vi "Check If Line Exists.vi"(8 "error in":errorcluster, 10 "Name to Locate":string, 11 "SQLite configuration in":refnum<class "SQLite configuration.lvclass">) -> (0 "error out":errorcluster, 1 "Index":i32, 2 "Line out":T1, 3 "SQLite configuration out":refnum<class "SQLite configuration.lvclass">, 5 "Found?":bool)   [LabVIEW 2014, in "SQLite configuration.lvclass"]
doc: "Checks if a line already exists within a configuration."
uses:
  SQLite configuration.lvclass
  Line.ctl
  <vilib>/NI/Tag Bus Module Framework/channel/TBM channel.lvclass
  SQLite configuration.lvclass/SQLite configuration.ctl
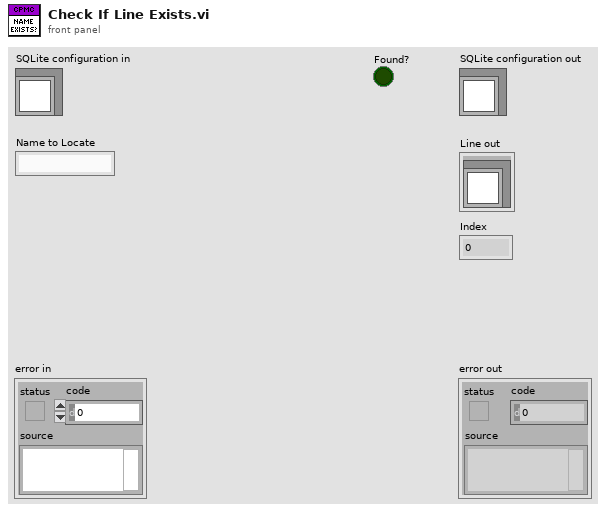
[diagram p1: front panel]
types:
  T1 = typedef "SQLite configuration.lvclass/Line.ctl" = cluster{"channel":refnum<class "TBM channel.lvclass">}
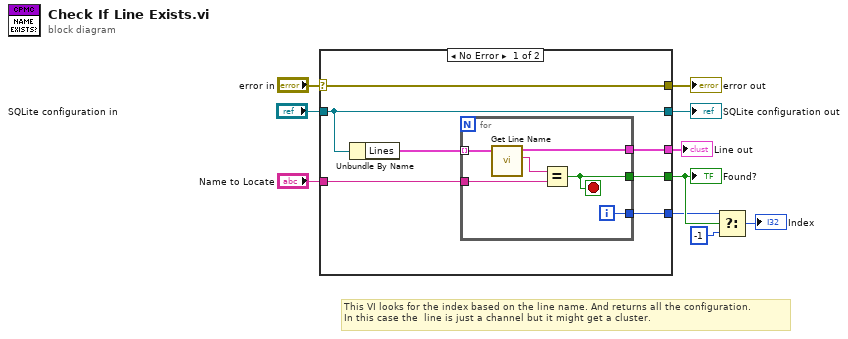
[diagram p0: block diagram]
diagram:
  # "This VI looks for the index based on the line name. And returns all the configuration. \nIn this case the  line is just a channel but it might get a cluster."
  n1 = case shown="No Error" "error in" {
    selector: "error in" -> [w17 w25]
    tunnel: [w17 w25] -> w9
    tunnel: [w16 w24] -> w7
    tunnel: "SQLite configuration in" -> [w16 w24]
    tunnel: "Name to Locate" -> [w14 _]
    tunnel: [w13 _] -> w3
    tunnel: [w12 _] -> w2
    tunnel: [w11 _] -> w1
    frame No Error {
      n2 = Unbundle By Name(w16) -> ("Lines"=w15:T1[])
      n3 = for {
        tunnel: w15 -> [w20] mode=indexing
        tunnel: w14 -> [w23]
        tunnel: [w22] -> w13
        tunnel: [w21] -> w12
        tunnel: [w18] -> w11
        i -> [w21]
        stop <- w22 stop-if-true
        n4 = call "Get Line Name.vi"("Line in"=w20) -> ("Name"=w19:string, "Line out"=w18:T1)  [unwired: 8 in, 1 out]
        n5 = Equal?(x=w19, y=w23) -> (x = y?=w22:bool)
      }
    }
    frame Error {
    }
  }
  "error out" <- w9
  "SQLite configuration out" <- w7
  "Found?" <- w3
  "Line out" <- w1
  n6 = Select(t=w2, s=w3, f=-1) -> (s? t:f=→"Index":i32)
